vi "FGEN Start Generator.vi"(8 "error in (no error)":errorcluster, 11 "Function Generator in":refnum<class "Function Generator.lvclass">) -> (0 "error out":errorcluster, 3 "Function Generator out":refnum<class "Function Generator.lvclass">)   [LabVIEW 2023, in "HardwareAbstractionLayer_LVOOP.lvlib" / "Function Generator.lvclass"]
uses:
  Function Generator.lvclass
  Function Generator.lvclass/Function Generator.ctl
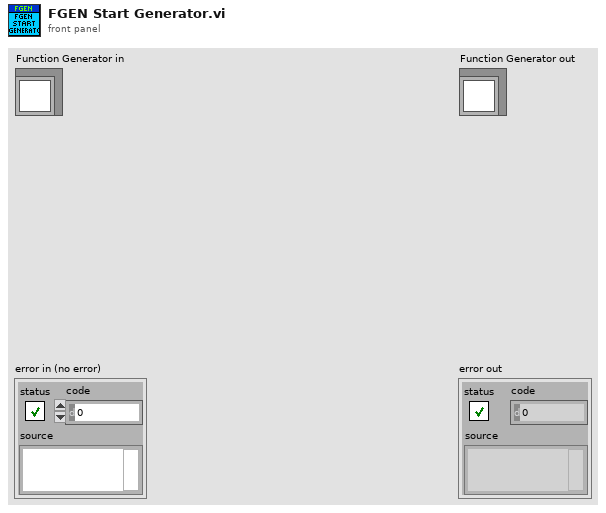
[diagram p1: front panel]
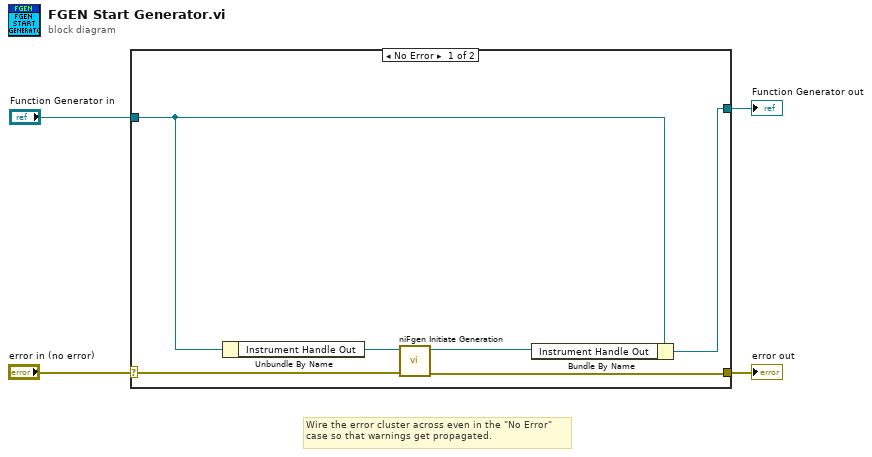
[diagram p0: block diagram]
diagram:
  # "Wire the error cluster across even in the \"No Error\"\ncase so that warnings get propagated."
  n1 = case shown="No Error" "error in (no error)" {
    selector: "error in (no error)" -> [w9 w12]
    tunnel: [w8 w12] -> w3
    tunnel: [w6 w11] -> w1
    tunnel: "Function Generator in" -> [w7 w11]
    frame No Error {
      n2 = Unbundle By Name(w7) -> ("Instrument Handle Out"=w10:refnum<k15>)
      n3 = call <instrlib>:"niFgen Initiate Generation.vi"("error in (no error)"=w9, "Instrument Handle"=w10) -> ("error out"=w8:errorcluster, "Instrument Handle Out"=w5:refnum<k15>)  [unwired: 8 in]
      n4 = Bundle By Name(cluster=w7, "Instrument Handle Out"=w5) -> (w6:refnum<class "Function Generator.lvclass">)
    }
    frame Error {
    }
  }
  "error out" <- w3
  "Function Generator out" <- w1
